vi "AODuint642MHz.vi"(4 "In u64":u64) -> (1 "Out MHz":dbl)   [LabVIEW 2013]
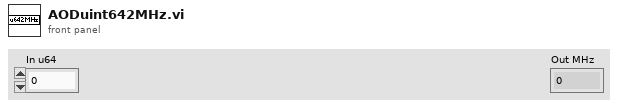
[diagram p1: front panel]
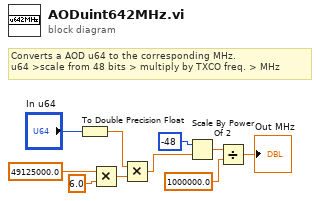
[diagram p0: block diagram]
diagram:
  # "Converts a AOD u64 to the corresponding MHz.\nu64 >scale from 48 bits > multiply by TXCO freq. > MHz"
  n1 = To Double Precision Float(number="In u64") -> (double precision float=w5:dbl)
  n2 = Multiply(x=49125000.0, y=6.0) -> (x*y=w6:dbl)
  n3 = Multiply(x=w5, y=w6) -> (x*y=w8:dbl)
  n4 = Scale By Power Of 2(n=-48, x=w8) -> (x*2^n=w9:dbl)
  n5 = Divide(x=w9, y=1000000.0) -> (x/y=→"Out MHz":dbl)
